vi "Intersection.vi"() -> ()   [LabVIEW 2023]
uses:
  <extravilib>/ChannelInstances/One Element Stream-u16/Read With Abort.vi
  <extravilib>/ChannelInstances/One Element Stream-u16/Instantiate.vi
  <extravilib>/ChannelInstances/One Element Stream-u16/EndpointRead.vi
  <extravilib>/ChannelInstances/One Element Stream-bool/Instantiate.vi
  <extravilib>/ChannelInstances/One Element Stream-u16.lvlib
panel:
  out "light":u16(ring)=2
  out "light":u16(ring)
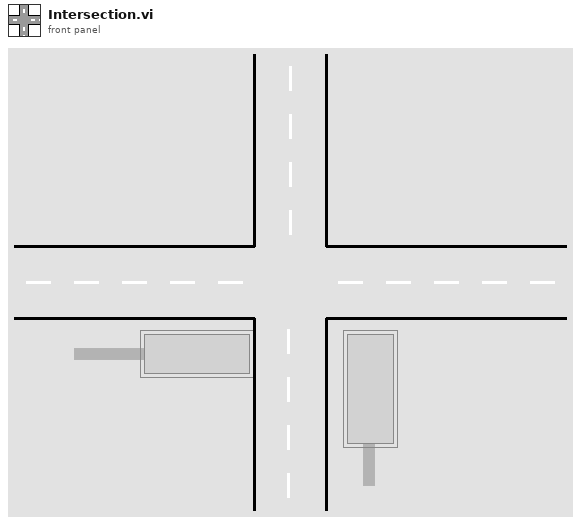
[diagram p1: front panel]
types:
  T1 = typedef "One Element Stream-u16.lvlib/)Channel.ctl" = refnum<queue>
  T2 = typedef "One Element Stream-bool.lvlib/)Channel.ctl" = refnum<queue>
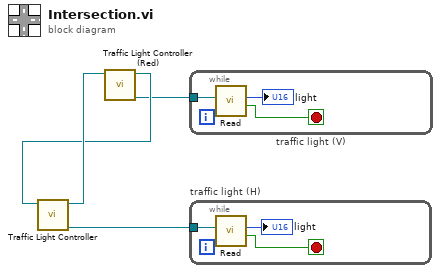
[diagram p0: block diagram]
diagram:
  n1 = call "Traffic Light Controller.vi"("peds stopped"=w2) -> ("traffic light"=w4:T1, "cars stopped"=w3:T2)  [unwired: 5 in]
  n2 = call "Traffic Light Controller (Red).vi"("peds stopped"=w3) -> ("traffic light"=w1:T1, "cars stopped"=w2:T2)  [unwired: 5 in]
  n3 = while "traffic light (V)" {
    tunnel: w1 -> [w7]
    stop <- w6 stop-if-true
    n4 = call <extravilib>:"Read.vi"("channel"=w7) -> ("last element?"=w6:bool, "element"=→"light":u16)  [unwired: 7 in, 2 out]
  }
  n5 = while "traffic light (H)" {
    tunnel: w4 -> [w10]
    stop <- w9 stop-if-true
    n6 = call <extravilib>:"Read.vi"("channel"=w10) -> ("last element?"=w9:bool, "element"=→"light":u16)  [unwired: 7 in, 2 out]
  }
